vi "test_PhotonPoseEstimator_Common_Make_Field.vi"() -> (3 "AprilTagFieldLayout":T1 {"OriginPose3d"."Translation3d"."Z" format="%14.3f"; "OriginPose3d"."Translation3d"."Y" format="%14.3f"; "OriginPose3d"."Translation3d"."X" format="%14.3f"})   [LabVIEW 2019]
uses:
  <vilib>/Rock Robotics/WPI/ThirdParty/JAS_Junk/TrajLib/Trajectory_Library.lvlib
  <vilib>/Rock Robotics/WPI/ThirdParty/JAS_Junk/TrajLib/TypeDef/TRANSLATION3D.ctl
  <vilib>/Rock Robotics/WPI/ThirdParty/JAS_Junk/TrajLib/TypeDef/QUATERNION.ctl
  <vilib>/Rock Robotics/WPI/ThirdParty/JAS_Junk/TrajLib/TypeDef/ROTATION3D.ctl
  <vilib>/Rock Robotics/WPI/ThirdParty/JAS_Junk/TrajLib/TypeDef/POSE3D.ctl
  <vilib>/Rock Robotics/WPI/ThirdParty/JAS_Junk/TrajLib/TypeDef/AprilTag.ctl
  <vilib>/Rock Robotics/WPI/ThirdParty/JAS_Junk/TrajLib/Enum/AprilTagFieldLayoutOrignPosition_ENUM.ctl
  <vilib>/Rock Robotics/WPI/ThirdParty/JAS_Junk/TrajLib/TypeDef/AprilTagFieldLayout.ctl
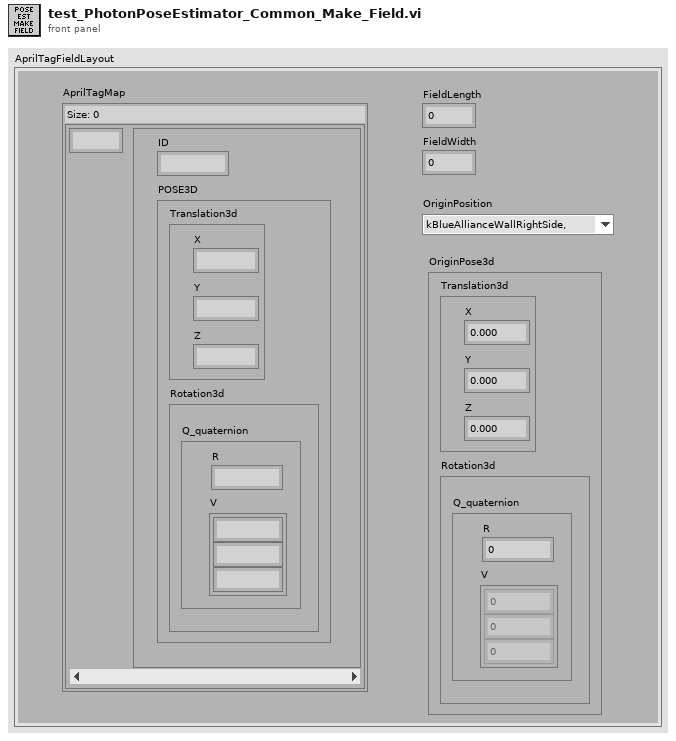
[diagram p1: front panel]
types:
  T1 = typedef "Trajectory_Library.lvlib/AprilTagFieldLayout.ctl" = cluster{"AprilTagMap":map{i32, T2}, "FieldLength":dbl, "FieldWidth":dbl, "OriginPosition ":T7, "OriginPose3d":T3}
  T2 = typedef "Trajectory_Library.lvlib/AprilTag.ctl" = cluster{"ID":i32, "POSE3D":T3}
  T3 = typedef "Trajectory_Library.lvlib/POSE3D.ctl" = cluster{"Translation3d":T4, "Rotation3d":T5}
  T4 = typedef "Trajectory_Library.lvlib/TRANSLATION3D.ctl" = cluster{"X":dbl, "Y":dbl, "Z":dbl}
  T5 = typedef "Trajectory_Library.lvlib/ROTATION3D.ctl" = cluster{"Q_quaternion":T6}
  T6 = typedef "Trajectory_Library.lvlib/QUATERNION.ctl" = cluster{"R":dbl, "V":dbl[]}
  T7 = typedef "Trajectory_Library.lvlib/AprilTagFieldLayoutOrignPosition_ENUM.ctl" = enum16{"kBlueAllianceWallRightSide,", "kRedAllianceWallRightSide,"}
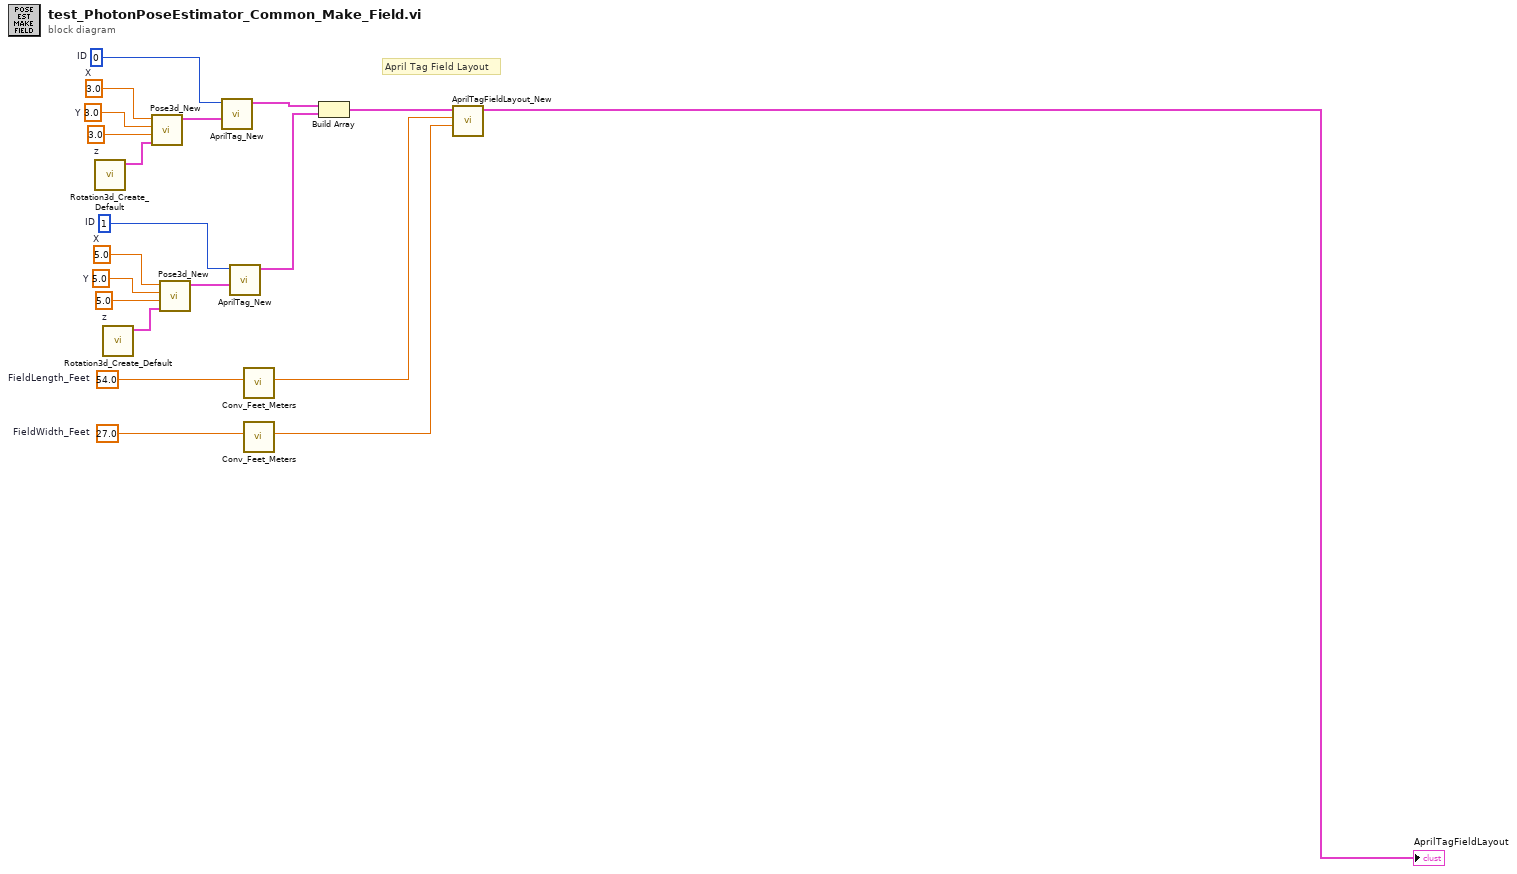
[diagram p0: block diagram]
diagram:
  w18 = 54.0  # FieldLength_Feet
  w19 = 27.0  # FieldWidth_Feet
  w11 = 5.0  # X
  w10 = 5.0  # Y
  w9 = 5.0  # z
  w7 = 1  # ID
  w5 = 3.0  # X
  w4 = 3.0  # Y
  w3 = 3.0  # z
  w1 = 0  # ID
  # "April Tag Field Layout"
  n1 = call <vilib>:"Rotation3d_Create_Default.vi"() -> ("ROTATION3D"=w2:T5)  [unwired: 11 in]
  n2 = call <vilib>:"Rotation3d_Create_Default.vi"() -> ("ROTATION3D"=w8:T5)  [unwired: 11 in]
  n3 = call <vilib>:"Pose3d_New.vi"("Rotation3d"=w2, "z"=w3, "Y"=w4, "X"=w5) -> ("out Pose3d"=w6:T3)  [unwired: 7 in]
  n4 = call <vilib>:"Pose3d_New.vi"("Rotation3d"=w8, "z"=w9, "Y"=w10, "X"=w11) -> ("out Pose3d"=w12:T3)  [unwired: 7 in]
  n5 = call <vilib>:"AprilTag_New.vi"("POSE3D"=w6, "ID"=w1) -> ("AprilTag"=w13:T2)  [unwired: 9 in]
  n6 = call <vilib>:"AprilTag_New.vi"("POSE3D"=w12, "ID"=w7) -> ("AprilTag"=w14:T2)  [unwired: 9 in]
  n7 = call <vilib>:"Conv_Feet_Meters.vi"("Feet"=w18) -> ("Meters"=w16:dbl)  [unwired: 10 in]
  n8 = call <vilib>:"Conv_Feet_Meters.vi"("Feet"=w19) -> ("Meters"=w17:dbl)  [unwired: 10 in]
  n9 = Build Array(w13, w14) -> (w15:T2[])
  n10 = call <vilib>:"AprilTagFieldLayout_New.vi"("FieldWidth_Meters"=w17, "FieldLength_Meters"=w16, "AprilTags"=w15) -> ("AprilTagFieldLayout"=→"AprilTagFieldLayout":T1)  [unwired: 8 in]
